vi "(Global) Extract-image and Results.vi"() -> ()   [LabVIEW 2014]
panel:
  in  "Results":dbl[](array[numeric])
  out "Image Extrace":T1(plugin-control)
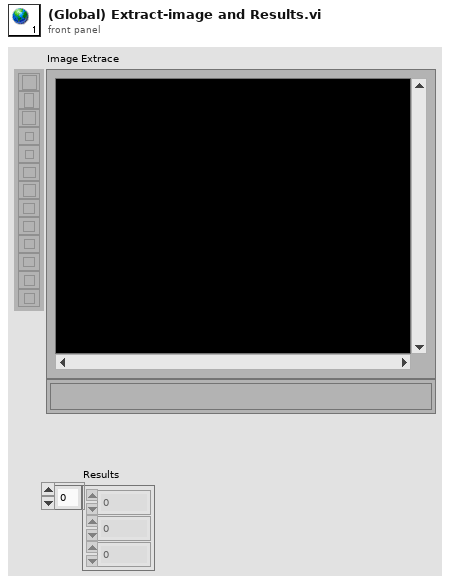
[diagram p1: front panel]
types:
  T1 = typedef "IMAQ Image.ctl" = refnum<image>
diagram:
